vi "GetServerNiceName.vi"(0 "ROS":T1, 1 "Text to add":string) -> (2 "String":string)   [LabVIEW 2012]
uses:
  <userlib>/ROSforLV/ROS/Code/SubVIs/_ROSControl.ctl
  <userlib>/ROSforLV/ROS/Code/SubVIs/_ROSDirection.ctl
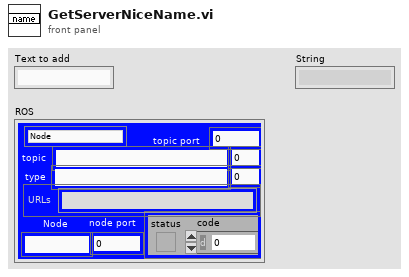
[diagram p1: front panel]
types:
  T1 = typedef "_ROSControl.ctl" = cluster{"topic port":u16, "Node":string, "topic":string, "type":string, "node port":u16, "error ":errorcluster, "Direction":T2, "APIs":string[], "Update (ms)":u16, "write queue":u16}
  T2 = typedef "_ROSDirection.ctl" = enum16{"Node", "Publisher", "Subscriber", "Service Client"}
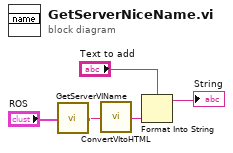
[diagram p0: block diagram]
diagram:
  n1 = call <userlib>:"GetServerVIName.vi"("ROS"="ROS") -> ("vi name"=w3:string)
  n2 = call <userlib>:"ConvertVItoHTML.vi"("vi name"=w3) -> ("Server Name"=w5:string)  [unwired: 1 out]
  n3 = Format Into String(format string="Text to add", w5) -> (resulting string=→"String":string)  [unwired: 2 in, 1 out]
